vi "LV SCISDK Add New Device.vi"(6 "handle":u64, 7 "Name":string, 8 "error in (no error)":errorcluster, 9 "JSONFwFilePath":string, 10 "DeviceModel":string, 11 "DevicePath":string) -> (0 "error out":errorcluster, 3 "function return":i32, 4 "handle out":u64)   [LabVIEW 2021, in "SciSDK_Labview.lvlib"]
doc: "You need this VI to call the native dll method to attach a device"
uses:
  SciSDK_Labview.lvlib
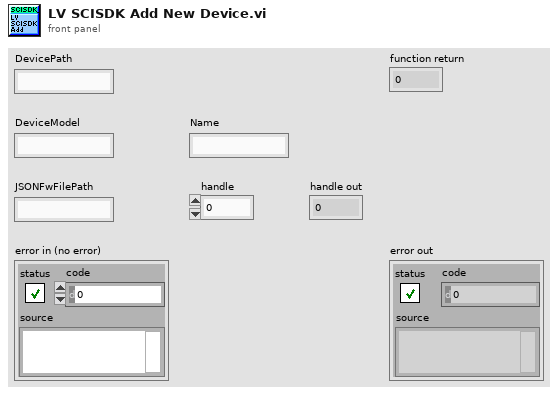
[diagram p1: front panel]
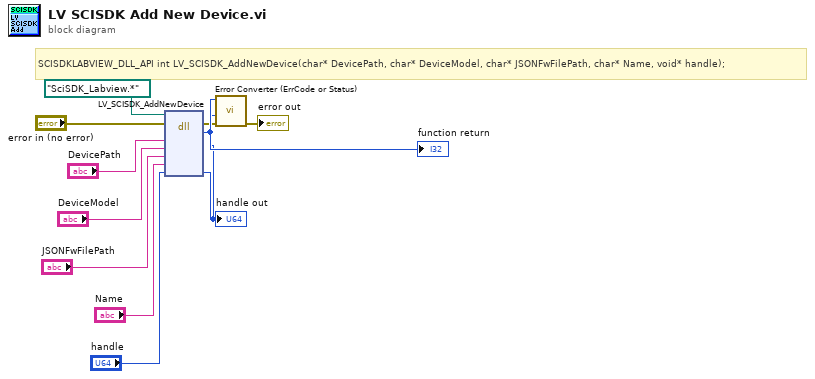
[diagram p0: block diagram]
diagram:
  # "SCISDKLABVIEW_DLL_API int LV_SCISDK_AddNewDevice(char* DevicePath, char* DeviceModel, char* JSONFwFilePath, char* Name, void* handle);"
  n1 = dll-call lib="C:/git/scisdk/bin/x64/Release/SciSDK_Labview.dll" fn="LV_SCISDK_AddNewDevice"(path in=path "SciSDK_Labview.*", error in="error in (no error)", "DevicePath"="DevicePath", "DeviceModel"="DeviceModel", "JSONFwFilePath"="JSONFwFilePath", "Name"="Name", "handle"="handle") -> (error out=w4:errorcluster, "return type"=w11:i32, "handle"=w1:u64)  [unwired: 5 in, 1 out]
  "function return" <- w11
  "handle out" <- w1
  n2 = call "Error Converter (ErrCode or Status).vi"("error in (no error)"=w4, "handle"=w1, "error code"=w11) -> ("error out"=→"error out":errorcluster)  [unwired: 8 in]
